vi "Agilent SNA Sort Measurements.vi"(7 "Agilent SNA & SWP":T7, 8 "error in (no error)":errorcluster, 9 "Auto Select":bool, 10 "Parameters to Measure":T1[](array[typedef]) {"Channel" min=1 max=99 step=1; "Parameter"."Stimulus Port" min=1 step=1; "Parameter"."Response Port" min=1 step=1}, 11 "VISA Resource Names":T5) -> (0 "error out":errorcluster {"code" format="%.0x"}, 1 "Channels Used":i8[](array[numeric]), 2 "Sorted Measurements":cluster{"Measurements":T6[]}[](array[cluster]) {"Measurements"."Traces"."Parameter"."Stimulus Port" min=1 step=1; "Measurements"."Traces"."Parameter"."Response Port" min=1 step=1}, 3 "dup VISA Resource Names":T5, 4 "Sorted Parameters to Measure":T1[](array[typedef]) {"Channel" min=1 max=99 step=1; "Parameter"."Stimulus Port" min=1 step=1; "Parameter"."Response Port" min=1 step=1}, 5 "Removed Parameters":T1[](array[typedef]) {"Channel" min=1 max=99 step=1; "Parameter"."Stimulus Port" min=1 step=1; "Parameter"."Response Port" min=1 step=1}, 6 "Measurements Removed?":bool)   [LabVIEW 2011]
uses:
  tests/S Parameter/TypeDefs/SP Parameter to Measure.ctl
  tests/S Parameter/TypeDefs/SP Parameter.ctl
  tests/S Parameter/TypeDefs/SP Calibration State.ctl
  tests/S Parameter/TypeDefs/SP Measurement Format.ctl
  TypeDefs/Agilent SNA Instrument Info.ctl
  TypeDefs/Agilent SNA Measurements.ctl
  TypeDefs/Agilent SNA VISA.ctl
  SI.LIB/Add to Array if Not Present (I32).vi
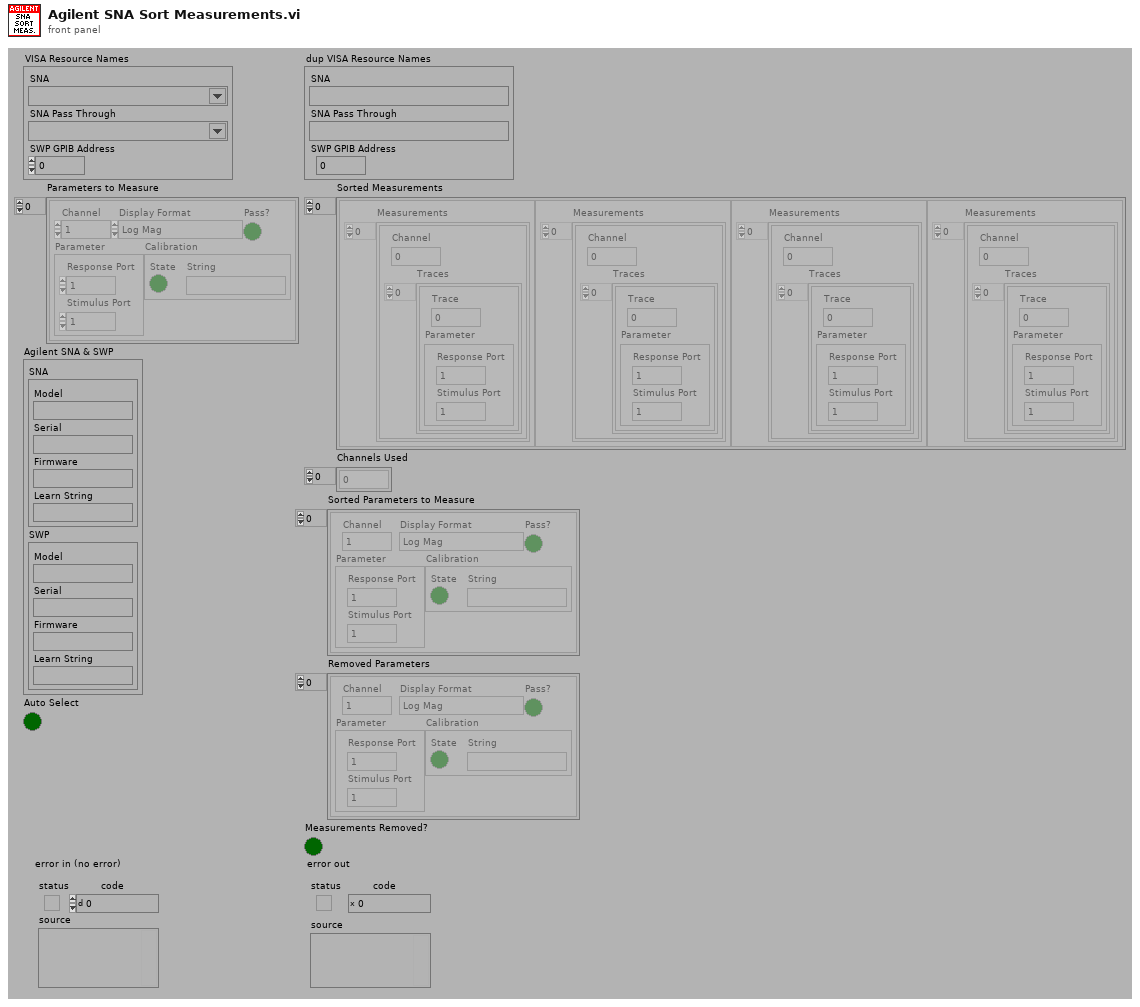
[diagram p1: front panel]
types:
  T1 = typedef "SP Parameter to Measure.ctl" = cluster{"Channel":i8, "Parameter":T2, "Calibration":T3, "Display Format":T4, "Pass?":bool}
  T2 = typedef "SP Parameter.ctl" = cluster{"Stimulus Port":i8, "Response Port":i8}
  T3 = typedef "SP Calibration State.ctl" = cluster{"State":bool, "String":string}
  T4 = typedef "SP Measurement Format.ctl" = enum32{"Log Mag", "Phase", "Delay", "Smith (R+jX)", "Polar (Re/Im)", "Linear Mag", "SWR", "Real", "Imaginary", "Smith (Lin/Phase)", "Smith (Log/Phase)", "Smith (Real/Imag)", "Smith (G+jB)", "Polar (Lin/Phase)", "Polar (Log/Phase)", "Expanded Phase", "Positive Phase", "Inverted Smith", "Unwrapped Phase", "Power Out", "Power In", "Linear Mag/Phase", "Log Mag/Phase", "Real/Imaginary"}
  T5 = typedef "Agilent SNA VISA.ctl" = cluster{"SNA":refnum<visa-resource-name>, "SNA Pass Through":refnum<visa-resource-name>, "SWP GPIB Address":i32}
  T6 = typedef "Agilent SNA Measurements.ctl" = cluster{"Channel":i8, "Traces":cluster{"Trace":i8, "Parameter":T2}[]}
  T7 = typedef "Agilent SNA Instrument Info.ctl" = cluster{"SNA":cluster{"Model":string, "Serial":string, "Firmware":string, "Learn String":string}, "SWP":cluster{"Model":string, "Serial":string, "Firmware":string, "Learn String":string}}
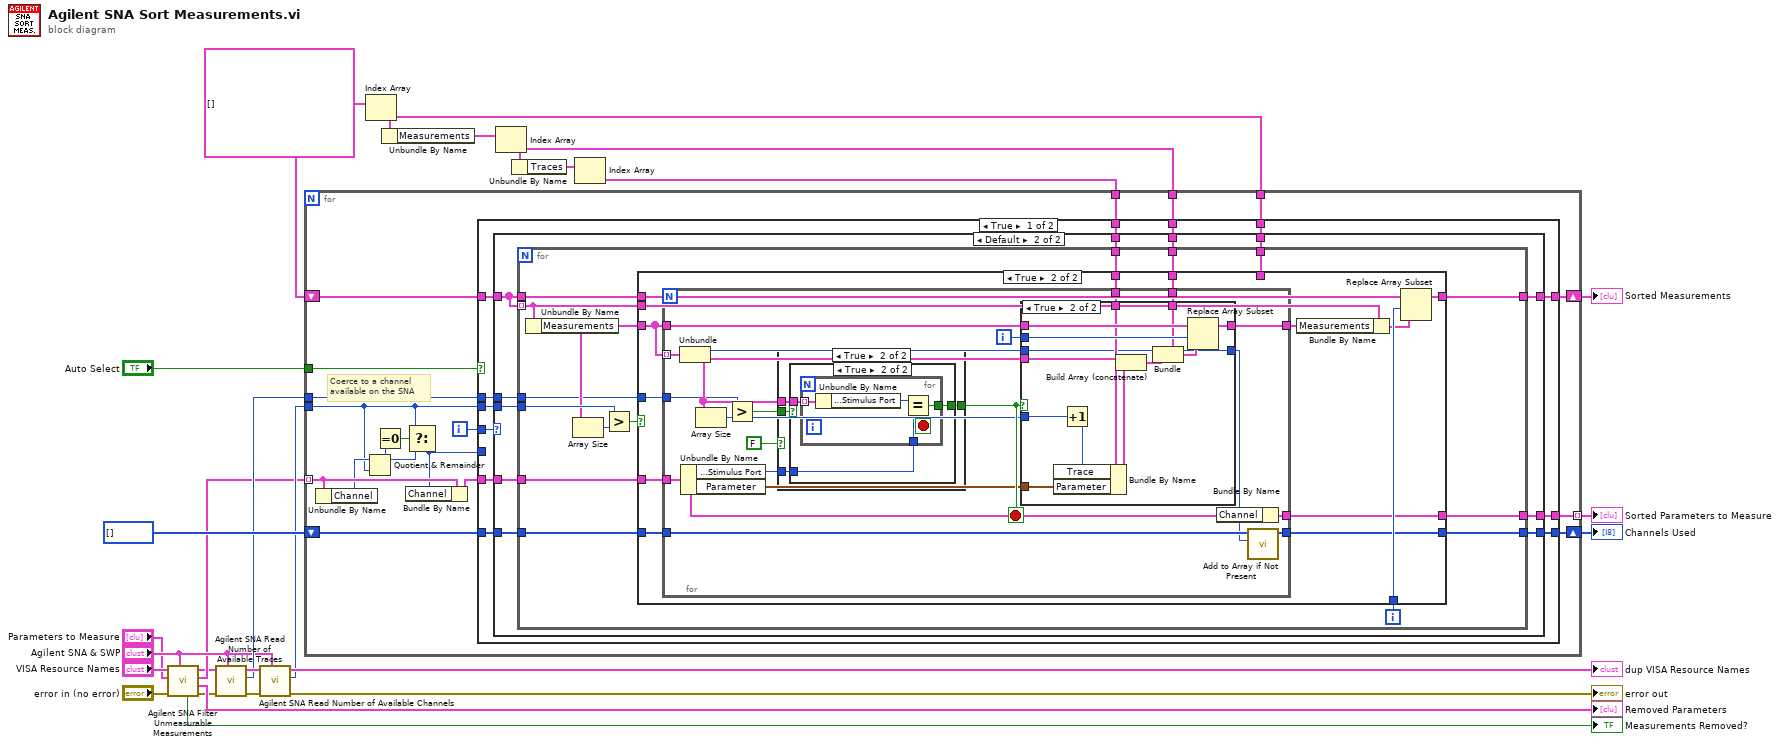
[diagram p0: block diagram]
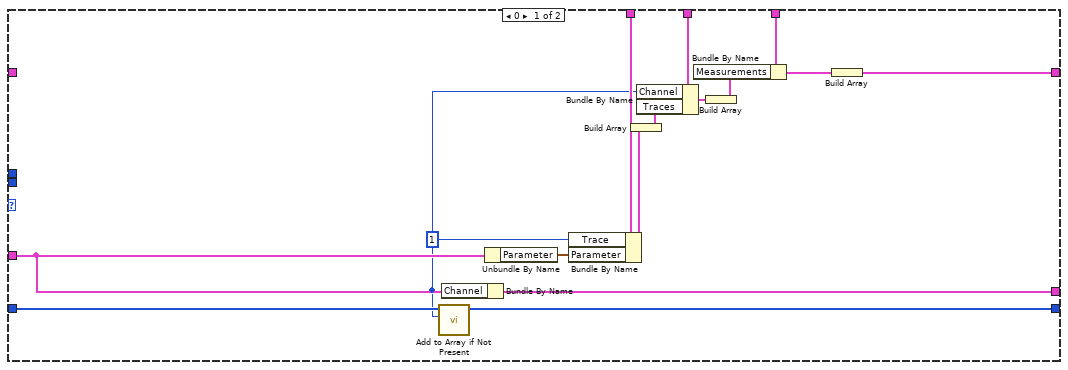
[diagram p2: hidden frame]
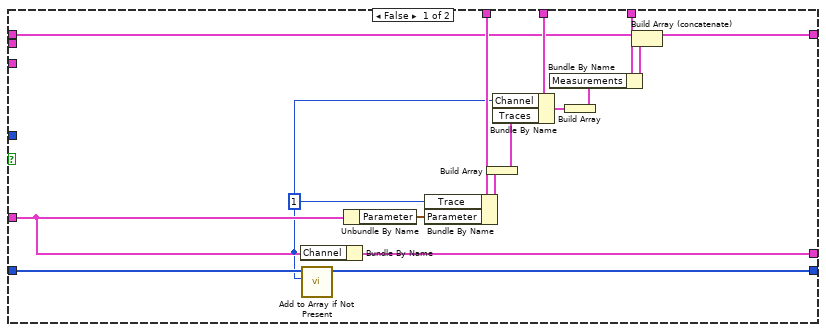
[diagram p3: hidden frame]
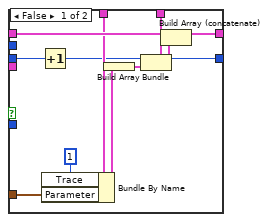
[diagram p6: hidden frame]
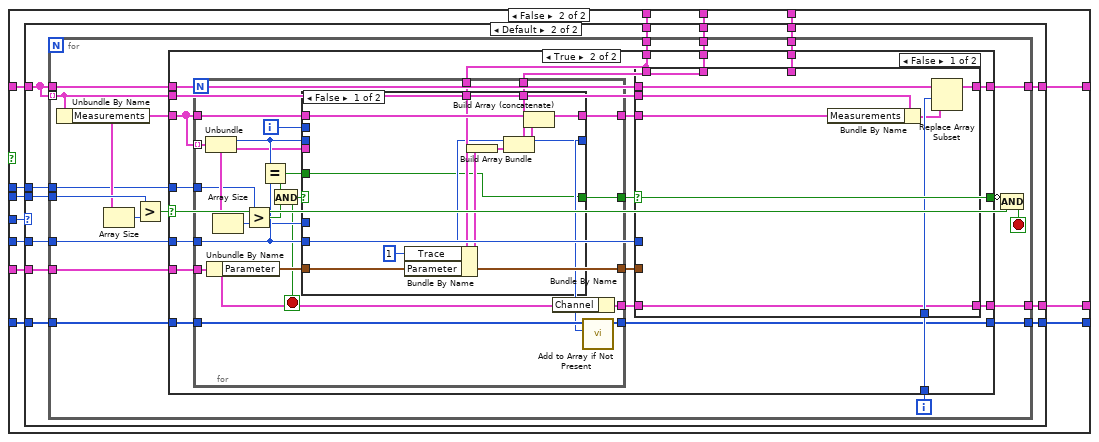
[diagram p7: hidden frame]
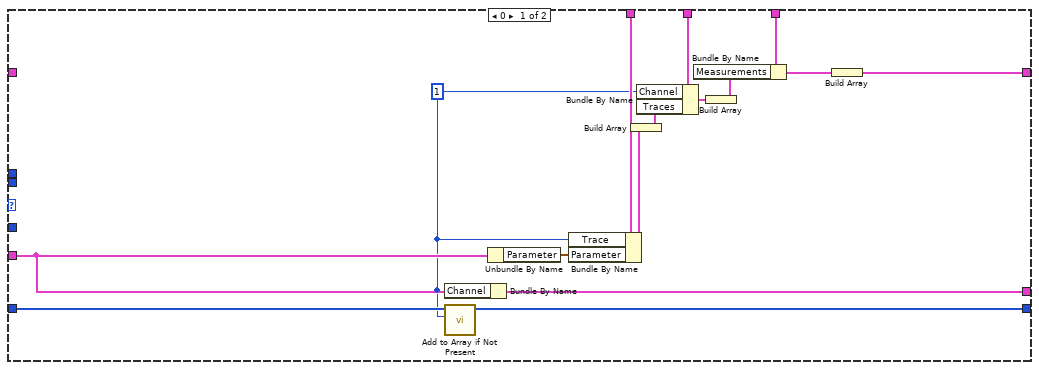
[diagram p8: hidden frame]
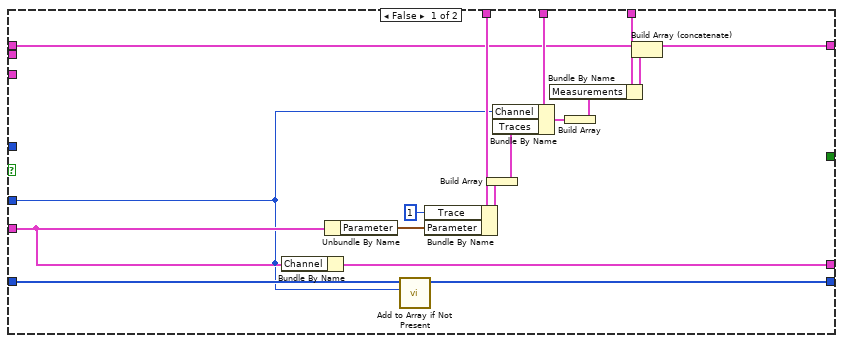
[diagram p9: hidden frame]
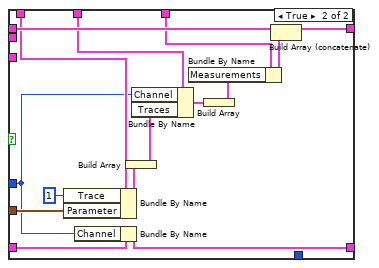
[diagram p10: hidden frame]
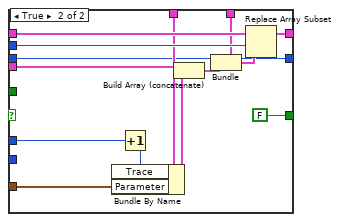
[diagram p11: hidden frame]
diagram:
  w21 = cluster{"Measurements":T6[]}[] [] ("Sorted Measurements")
  n1 = call "Agilent SNA Filter Unmeasurable Measurements.vi"("Agilent SNA & SWP"="Agilent SNA & SWP", "error in (no error)"="error in (no error)", "Parameters to Measure"="Parameters to Measure", "VISA Resource Names"="VISA Resource Names") -> ("error out"=w1:errorcluster, "Removed Parameters"=→"Removed Parameters":T1[], "Filtered Parameters to Measure"=w6:T1[], "dup VISA Resource Names"=w2:T5, "Measurements Removed?"=→"Measurements Removed?":bool)  [unwired: 3 out]
  n2 = call "Agilent SNA Read Number of Available Traces.vi"("Agilent SNA & SWP"="Agilent SNA & SWP", "error in (no error)"=w1, "VISA Resource Names"=w2) -> ("error out"=w13:errorcluster, "Number of Traces"=w11:i8, "dup VISA Resource Names"=w12:T5)  [unwired: 6 out]
  n3 = call "Agilent SNA Read Number of Available Channels.vi"("Agilent SNA & SWP"="Agilent SNA & SWP", "error in (no error)"=w13, "VISA Resource Names"=w12) -> ("error out"=→"error out":errorcluster, "Number of Channels"=w14:i8, "dup VISA Resource Names"=→"dup VISA Resource Names":T5)  [unwired: 6 out]
  n4 = Index Array(array=w21) -> (element=w17:cluster{"Measurements":T6[]})  [unwired: 1 in]
  n5 = Unbundle By Name(w17) -> ("Measurements"=w23:T6[])
  n6 = Index Array(array=w23) -> (element=w18:T6)  [unwired: 1 in]
  n7 = Unbundle By Name(w18) -> ("Traces"=w20:cluster{"Trace":i8, "Parameter":T2}[])
  n8 = Index Array(array=w20) -> (element=w19:cluster{"Trace":i8, "Parameter":T2})  [unwired: 1 in]
  n9 = for {
    tunnel: w6 -> [w42] mode=indexing
    shift-right: [w32] -> w22
    shift-left: w21 -> [w43]
    tunnel: w14 -> [w37]
    tunnel: "Auto Select" -> [w35]
    tunnel: w19 -> [w34]
    tunnel: w18 -> [w33]
    tunnel: w17 -> [w31]
    shift-right: [w29] -> w15
    shift-left: i8[] [] -> [w30]
    tunnel: w11 -> [w28]
    tunnel: [w27] -> w5 mode=indexing
    i -> [w44]
    # "Coerce to a channel\navailable on the SNA"
    n10 = Unbundle By Name(w42) -> ("Channel"=w40:i8)
    n11 = Quotient & Remainder(x=w40, y=w37) -> (x-y*floor(x/y)=w36:i8)  [unwired: 1 out]
    n12 = Equal To 0?(x=w36) -> (x = 0?=w39:bool)
    n13 = Select(t=w37, s=w39, f=w36) -> (s? t:f=w38:i8)
    n14 = Bundle By Name(cluster=w42, "Channel"=w38) -> (w41:T1)
    n15 = case shown="True" w35 {
      tunnel: w44 -> [w50 w192]
      tunnel: w43 -> [w56 w198]
      tunnel: w41 -> [w55 w197]
      tunnel: w38 -> [_ w188]
      tunnel: w37 -> [w54 w196]
      tunnel: w34 -> [w53 w195]
      tunnel: w33 -> [w52 w194]
      tunnel: [w51 w193] -> w32
      tunnel: w31 -> [w49 w191]
      tunnel: w30 -> [w48 w190]
      tunnel: [w47 w189] -> w29
      tunnel: w28 -> [w46 w187]
      tunnel: [w45 w186] -> w27
      frame True {
        n16 = case shown="Default" w50 {
          tunnel: w56 -> [_ w77]
          tunnel: w55 -> [w59 w82]
          tunnel: w54 -> [_ w81]
          tunnel: w53 -> [w71 w80]
          tunnel: w52 -> [w69 w79]
          tunnel: [w62 w78] -> w51
          tunnel: w49 -> [w65 w76]
          tunnel: w48 -> [w61 w75]
          tunnel: [w60 w74] -> w47
          tunnel: w46 -> [_ w73]
          tunnel: [w57 w72] -> w45
          frame 0 {
            w58 = i8 1 ("Trace")
            n17 = call-poly "Add to Array if Not Present.vi"("I32"=w58, "I32 Array"=w61) -> ("New I32 Array"=w60:i32[])  [unwired: 3 out]
            n18 = Bundle By Name(cluster=w59, "Channel"=w58) -> (w57:T1)
            n19 = Unbundle By Name(w59) -> ("Parameter"=w70:T2)
            n20 = Bundle By Name(cluster=w71, "Trace"=w58, "Parameter"=w70) -> (w67:cluster{"Trace":i8, "Parameter":T2})
            n21 = Build Array(w67) -> (w66:cluster{"Trace":i8, "Parameter":T2}[])
            n22 = Bundle By Name(cluster=w69, "Channel"=w58, "Traces"=w66) -> (w68:T6)
            n23 = Build Array(w68) -> (w64:T6[])
            n24 = Bundle By Name(cluster=w65, "Measurements"=w64) -> (w63:cluster{"Measurements":T6[]})
            n25 = Build Array(w63) -> (w62:cluster{"Measurements":T6[]}[])
          }
          frame Default {
            n26 = for {
              tunnel: w77 -> [w91]
              tunnel: w82 -> [w98]
              tunnel: w81 -> [w94]
              tunnel: w80 -> [w97]
              tunnel: w79 -> [w96]
              tunnel: [w95] -> w78
              tunnel: w77 -> [w87] mode=indexing
              tunnel: w76 -> [w88]
              tunnel: w75 -> [w86]
              tunnel: [w85] -> w74
              tunnel: w73 -> [w84]
              tunnel: [w83] -> w72
              i -> [w90]
              n27 = Unbundle By Name(w87) -> ("Measurements"=w89:T6[])
              n28 = Array Size(array=w89) -> (size(s)=w93:i32)
              n29 = Greater?(x=w94, y=w93) -> (0:w92:bool)
              n30 = case shown="True" w92 {
                tunnel: w98 -> [w101 w128]
                tunnel: w97 -> [w112 w127]
                tunnel: w96 -> [w111 w126]
                tunnel: [w114 w123] -> w95
                tunnel: w89 -> [_ w125]
                tunnel: w91 -> [w108 w124]
                tunnel: w90 -> [_ w122]
                tunnel: w88 -> [w106 _]
                tunnel: w87 -> [_ w121]
                tunnel: w86 -> [w103 w118]
                tunnel: [w102 w117] -> w85
                tunnel: w84 -> [_ w116]
                tunnel: [w100 w115] -> w83
                frame False {
                  w99 = i8 1 ("Channel")
                  n31 = Bundle By Name(cluster=w101, "Channel"=w99) -> (w100:T1)
                  n32 = call-poly "Add to Array if Not Present.vi"("I32"=w99, "I32 Array"=w103) -> ("New I32 Array"=w102:i32[])  [unwired: 3 out]
                  n33 = Unbundle By Name(w101) -> ("Parameter"=w113:T2)
                  n34 = Bundle By Name(cluster=w112, "Trace"=w99, "Parameter"=w113) -> (w110:cluster{"Trace":i8, "Parameter":T2})
                  n35 = Build Array(w110) -> (w109:cluster{"Trace":i8, "Parameter":T2}[])
                  n36 = Bundle By Name(cluster=w111, "Channel"=w99, "Traces"=w109) -> (w107:T6)
                  n37 = Build Array(w107) -> (w105:T6[])
                  n38 = Bundle By Name(cluster=w106, "Measurements"=w105) -> (w104:cluster{"Measurements":T6[]})
                  n39 = Build Array (concatenate)(w108, w104) -> (w114:cluster{"Measurements":T6[]}[])
                }
                frame True {
                  n40 = for {
                    tunnel: w125 -> [w144] mode=indexing
                    tunnel: w128 -> [w132]
                    tunnel: w125 -> [w148]
                    tunnel: [w145] -> w120
                    tunnel: w127 -> [w140]
                    tunnel: w126 -> [w138]
                    tunnel: w118 -> [w135]
                    tunnel: [w134] -> w117
                    tunnel: w116 -> [w133]
                    tunnel: [w131] -> w115
                    i -> [w147]
                    stop <- w143 stop-if-true
                    n41 = Unbundle(w144) -> ("Channel"=w141:i8, "Traces"=w142:cluster{"Trace":i8, "Parameter":T2}[])
                    n42 = Unbundle By Name(w132) -> ("Parameter.Stimulus Port"=w136:i8, "Parameter"=w137:T2)
                    n43 = Array Size(array=w142) -> (size(s)=w139:i32)
                    n44 = Greater?(x=w133, y=w139) -> (0:w146:bool)
                    n45 = case shown="True" FALSE {
                      tunnel: w146 -> [w149 w153]
                      tunnel: [w149 w152] -> w143
                      tunnel: w142 -> [_ w151]
                      tunnel: w136 -> [_ w150]
                      frame False {
                        # "We are no longer sorting by\nstimulus port.  We have decided\nthat it is no faster since it has to\nsweep once for each stimulus\nport no matter the configuration."
                      }
                      frame True {
                        n46 = case shown="True" w153 {
                          selector: w153 -> [w154 _]
                          tunnel: w151 -> [_ w157]
                          tunnel: [w154 w156] -> w152
                          tunnel: w150 -> [_ w155]
                          frame False {
                          }
                          frame True {
                            n47 = for {
                              tunnel: w157 -> [w161] mode=indexing
                              tunnel: [w159] -> w156
                              tunnel: w155 -> [w158]
                              stop <- w159 stop-if-true
                              n48 = Unbundle By Name(w161) -> ("Parameter.Stimulus Port"=w160:i8)
                              n49 = Equal?(x=w160, y=w158) -> (x = y?=w159:bool)
                            }
                          }
                        }
                      }
                    }
                    n50 = case shown="True" w143 {
                      tunnel: w142 -> [_ w181]
                      tunnel: w148 -> [w172 w185]
                      tunnel: w147 -> [_ w184]
                      tunnel: [w171 w183] -> w145
                      tunnel: w141 -> [w164 w173]
                      tunnel: w137 -> [w167 w179]
                      tunnel: w140 -> [w166 w180]
                      tunnel: w139 -> [_ w178]
                      tunnel: w138 -> [w168 w175]
                      tunnel: [w162 w173] -> w130
                      frame False {
                        n51 = Increment(x=w164) -> (x+1=w162:i8)
                        n52 = Bundle By Name(cluster=w166, "Trace"=i8 1, "Parameter"=w167) -> (w165:cluster{"Trace":i8, "Parameter":T2})
                        n53 = Build Array(w165) -> (w169:cluster{"Trace":i8, "Parameter":T2}[])
                        n54 = Bundle(cluster=w168, "Channel"=w162, "Traces"=w169) -> (w170:T6)
                        n55 = Build Array (concatenate)(w172, w170) -> (w171:T6[])
                      }
                      frame True {
                        n56 = Increment(x=w178) -> (x+1=w177:i32)
                        n57 = Bundle By Name(cluster=w180, "Trace"=w177, "Parameter"=w179) -> (w176:cluster{"Trace":i8, "Parameter":T2})
                        n58 = Build Array (concatenate)(w181, w176) -> (w174:cluster{"Trace":i8, "Parameter":T2}[])
                        n59 = Bundle(cluster=w175, "Channel"=w173, "Traces"=w174) -> (w182:T6)
                        n60 = Replace Array Subset(array=w185, new element=w182, index=w184) -> (w183:T6[])
                      }
                    }
                    n61 = Bundle By Name(cluster=w132, "Channel"=w130) -> (w131:T1)
                    n62 = call-poly "Add to Array if Not Present.vi"("I32"=w130, "I32 Array"=w135) -> ("New I32 Array"=w134:i32[])  [unwired: 3 out]
                  }
                  n63 = Bundle By Name(cluster=w121, "Measurements"=w120) -> (w119:cluster{"Measurements":T6[]})
                  n64 = Replace Array Subset(array=w124, new element=w119, index=w122) -> (w123:cluster{"Measurements":T6[]}[])
                }
              }
            }
          }
        }
      }
      frame False {
        n65 = case shown="Default" w192 {
          tunnel: w198 -> [_ w220]
          tunnel: w197 -> [w201 w225]
          tunnel: w196 -> [_ w224]
          tunnel: w195 -> [w213 w223]
          tunnel: w194 -> [w211 w222]
          tunnel: [w204 w221] -> w193
          tunnel: w191 -> [w207 w219]
          tunnel: w190 -> [w203 w218]
          tunnel: [w202 w217] -> w189
          tunnel: w188 -> [_ w216]
          tunnel: w187 -> [_ w215]
          tunnel: [w200 w214] -> w186
          frame 0 {
            w199 = i8 1 ("Channel")
            n66 = Bundle By Name(cluster=w201, "Channel"=w199) -> (w200:T1)
            n67 = call-poly "Add to Array if Not Present.vi"("I32"=w199, "I32 Array"=w203) -> ("New I32 Array"=w202:i32[])  [unwired: 3 out]
            n68 = Unbundle By Name(w201) -> ("Parameter"=w212:T2)
            n69 = Bundle By Name(cluster=w213, "Trace"=w199, "Parameter"=w212) -> (w209:cluster{"Trace":i8, "Parameter":T2})
            n70 = Build Array(w209) -> (w208:cluster{"Trace":i8, "Parameter":T2}[])
            n71 = Bundle By Name(cluster=w211, "Channel"=w199, "Traces"=w208) -> (w210:T6)
            n72 = Build Array(w210) -> (w206:T6[])
            n73 = Bundle By Name(cluster=w207, "Measurements"=w206) -> (w205:cluster{"Measurements":T6[]})
            n74 = Build Array(w205) -> (w204:cluster{"Measurements":T6[]}[])
          }
          frame Default {
            n75 = for {
              tunnel: w220 -> [w238]
              tunnel: w225 -> [w244]
              tunnel: w224 -> [w240]
              tunnel: w223 -> [w243]
              tunnel: w222 -> [w242]
              tunnel: [w241] -> w221
              tunnel: w220 -> [w234] mode=indexing
              tunnel: w219 -> [w235]
              tunnel: w218 -> [w233]
              tunnel: [w232] -> w217
              tunnel: w216 -> [w231]
              tunnel: w215 -> [w227]
              tunnel: [w226] -> w214
              i -> [w237]
              stop <- w228 stop-if-true
              n76 = Unbundle By Name(w234) -> ("Measurements"=w236:T6[])
              n77 = Array Size(array=w236) -> (size(s)=w239:i32)
              n78 = Greater?(x=w240, y=w239) -> (0:w229:bool)
              n79 = case shown="True" w229 {
                tunnel: w244 -> [w247 w279]
                tunnel: w243 -> [w259 w270]
                tunnel: w242 -> [w258 w269]
                tunnel: [w261 w276] -> w241
                tunnel: w236 -> [_ w278]
                tunnel: w238 -> [w255 w277]
                tunnel: w237 -> [_ w275]
                tunnel: w235 -> [w253 w266]
                tunnel: w234 -> [_ w274]
                tunnel: w233 -> [w250 w272]
                tunnel: [w249 w271] -> w232
                tunnel: w231 -> [w246 w267]
                tunnel: [_ w265] -> w230
                tunnel: w227 -> [_ w264]
                tunnel: [w245 w263] -> w226
                frame False {
                  n80 = Bundle By Name(cluster=w247, "Channel"=w246) -> (w245:T1)
                  n81 = Unbundle By Name(w247) -> ("Parameter"=w260:T2)
                  n82 = call-poly "Add to Array if Not Present.vi"("I32"=w246, "I32 Array"=w250) -> ("New I32 Array"=w249:i32[])  [unwired: 3 out]
                  n83 = Bundle By Name(cluster=w259, "Trace"=i8 1 ("Channel"), "Parameter"=w260) -> (w257:cluster{"Trace":i8, "Parameter":T2})
                  n84 = Build Array(w257) -> (w256:cluster{"Trace":i8, "Parameter":T2}[])
                  n85 = Bundle By Name(cluster=w258, "Channel"=w246, "Traces"=w256) -> (w254:T6)
                  n86 = Build Array(w254) -> (w252:T6[])
                  n87 = Bundle By Name(cluster=w253, "Measurements"=w252) -> (w251:cluster{"Measurements":T6[]})
                  n88 = Build Array (concatenate)(w255, w251) -> (w261:cluster{"Measurements":T6[]}[])
                }
                frame True {
                  n89 = for {
                    tunnel: w278 -> [w319] mode=indexing
                    tunnel: w279 -> [w304]
                    tunnel: w278 -> [w322]
                    tunnel: [w320] -> w273
                    tunnel: w270 -> [w318]
                    tunnel: w269 -> [w317]
                    tunnel: w272 -> [w316]
                    tunnel: [w315] -> w271
                    tunnel: w267 -> [w310]
                    tunnel: [w313] -> w268
                    tunnel: [w307] -> w265
                    tunnel: w264 -> [w305]
                    tunnel: [w302] -> w262
                    i -> [w321]
                    stop <- w308 stop-if-true
                    n90 = Unbundle(w319) -> ("Channel"=w314:i8, "Traces"=w312:cluster{"Trace":i8, "Parameter":T2}[])
                    n91 = Unbundle By Name(w304) -> ("Parameter"=w313:T2)
                    n92 = Array Size(array=w312) -> (size(s)=w309:i32)
                    n93 = Greater?(x=w305, y=w309) -> (0:w311:bool)
                    n94 = Equal?(x=w314, y=w310) -> (x = y?=w306:bool)
                    n95 = And(x=w306, y=w311) -> (x .and. y?=w308:bool)
                    n96 = case shown="False" w308 {
                      tunnel: w312 -> [_ w343]
                      tunnel: w322 -> [w333 w347]
                      tunnel: w321 -> [_ w346]
                      tunnel: [w332 w345] -> w320
                      tunnel: w314 -> [_ w337]
                      tunnel: w313 -> [w326 w341]
                      tunnel: w318 -> [w328 w342]
                      tunnel: w317 -> [w329 w339]
                      tunnel: [w324 w337] -> w303
                      tunnel: w310 -> [w324 _]
                      tunnel: w309 -> [_ w336]
                      tunnel: [w323 FALSE] -> w307
                      tunnel: w306 -> [w323 _]
                      frame False {
                        n97 = Bundle By Name(cluster=w328, "Trace"=i8 1, "Parameter"=w326) -> (w327:cluster{"Trace":i8, "Parameter":T2})
                        n98 = Build Array(w327) -> (w330:cluster{"Trace":i8, "Parameter":T2}[])
                        n99 = Bundle(cluster=w329, "Channel"=w324, "Traces"=w330) -> (w331:T6)
                        n100 = Build Array (concatenate)(w333, w331) -> (w332:T6[])
                      }
                      frame True {
                        n101 = Increment(x=w336) -> (x+1=w335:i32)
                        n102 = Bundle By Name(cluster=w342, "Trace"=w335, "Parameter"=w341) -> (w340:cluster{"Trace":i8, "Parameter":T2})
                        n103 = Build Array (concatenate)(w343, w340) -> (w338:cluster{"Trace":i8, "Parameter":T2}[])
                        n104 = Bundle(cluster=w339, "Channel"=w337, "Traces"=w338) -> (w344:T6)
                        n105 = Replace Array Subset(array=w347, new element=w344, index=w346) -> (w345:T6[])
                      }
                    }
                    n106 = Bundle By Name(cluster=w304, "Channel"=w303) -> (w302:T1)
                    n107 = call-poly "Add to Array if Not Present.vi"("I32"=w303, "I32 Array"=w316) -> ("New I32 Array"=w315:i32[])  [unwired: 3 out]
                  }
                  n108 = case shown="False" w265 {
                    tunnel: w277 -> [w286 w295]
                    tunnel: [w285 w294] -> w276
                    tunnel: w275 -> [w284 _]
                    tunnel: w274 -> [w283 _]
                    tunnel: w273 -> [w282 _]
                    tunnel: w270 -> [_ w293]
                    tunnel: w269 -> [_ w291]
                    tunnel: w268 -> [_ w292]
                    tunnel: w267 -> [_ w287]
                    tunnel: w266 -> [_ w290]
                    tunnel: [w280 w288] -> w263
                    tunnel: w262 -> [w280 w289]
                    frame False {
                      n109 = Bundle By Name(cluster=w283, "Measurements"=w282) -> (w281:cluster{"Measurements":T6[]})
                      n110 = Replace Array Subset(array=w286, new element=w281, index=w284) -> (w285:cluster{"Measurements":T6[]}[])
                    }
                    frame True {
                      n111 = Bundle By Name(cluster=w293, "Trace"=i8 1 ("Channel"), "Parameter"=w292) -> (w301:cluster{"Trace":i8, "Parameter":T2})
                      n112 = Bundle By Name(cluster=w289, "Channel"=w287) -> (w288:T1)
                      n113 = Build Array(w301) -> (w300:cluster{"Trace":i8, "Parameter":T2}[])
                      n114 = Bundle By Name(cluster=w291, "Channel"=w287, "Traces"=w300) -> (w299:T6)
                      n115 = Build Array(w299) -> (w298:T6[])
                      n116 = Bundle By Name(cluster=w290, "Measurements"=w298) -> (w297:cluster{"Measurements":T6[]})
                      n117 = Build Array (concatenate)(w295, w297) -> (w294:cluster{"Measurements":T6[]}[])
                    }
                  }
                }
              }
              n118 = Compound Arithmetic op=AND(invert w230, w229) -> (w228:bool)
            }
          }
        }
      }
    }
  }
  "Sorted Measurements" <- w22
  "Channels Used" <- w15
  "Sorted Parameters to Measure" <- w5
